vi "Pos.vi"() -> ()   [LabVIEW 2012]
panel:
  out "Y Pos":dbl
  out "X Pos":dbl
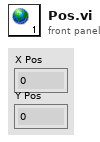
[diagram p1: front panel]
diagram:
